vi "price.vi"(11 "Path":path) -> (1 "result string":string, 2 "match substring":string, 3 "RESULT":string)   [LabVIEW 2018]
panel:
  in  "string":string="This will cost you : "
  in  "1":string="Yuu have selected "
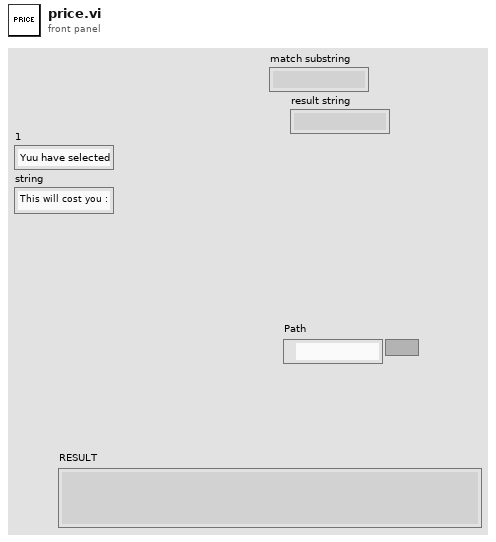
[diagram p1: front panel]
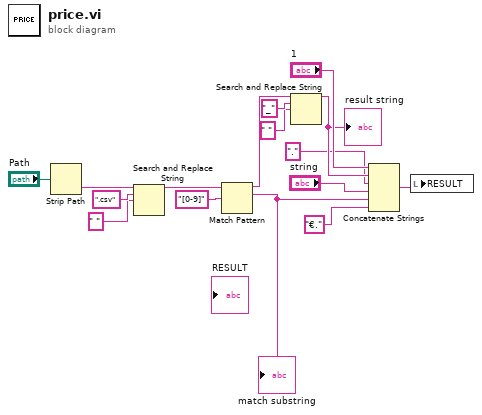
[diagram p0: block diagram]
diagram:
  n1 = Strip Path(path="Path") -> (name=w16:string)  [unwired: 1 out]
  n2 = Search and Replace String(input string=w16, search string=".csv", replace string=" " ("replace string (\"\")")) -> (result string=w10:string)  [unwired: 5 in, 3 out]
  n3 = Match Pattern(string=w10, regular expression="[0-9]") -> (before substring=w9:string, match substring=w3:string)  [unwired: 1 in, 2 out]
  "match substring" <- w3
  n4 = Search and Replace String(input string=w9, search string="_", replace string=" " ("replace string (\"\")")) -> (result string=w6:string)  [unwired: 5 in, 3 out]
  "result string" <- w6
  n5 = Concatenate Strings("1", w6, "." ("string"), "string", w3, "€." ("string")) -> (w11:string)
  n6 = local write "RESULT"(w11) -> ()
